vi "StateAlarmManagement.vi"(0 "Master State":enum16{"Normal", "Climb"}(ring)) -> ()   [LabVIEW 2020]
uses:
  sensordata.vi
  driverdata.vi
  autonomousinfo.vi
  robotoutputs.vi
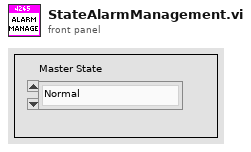
[diagram p1: front panel]
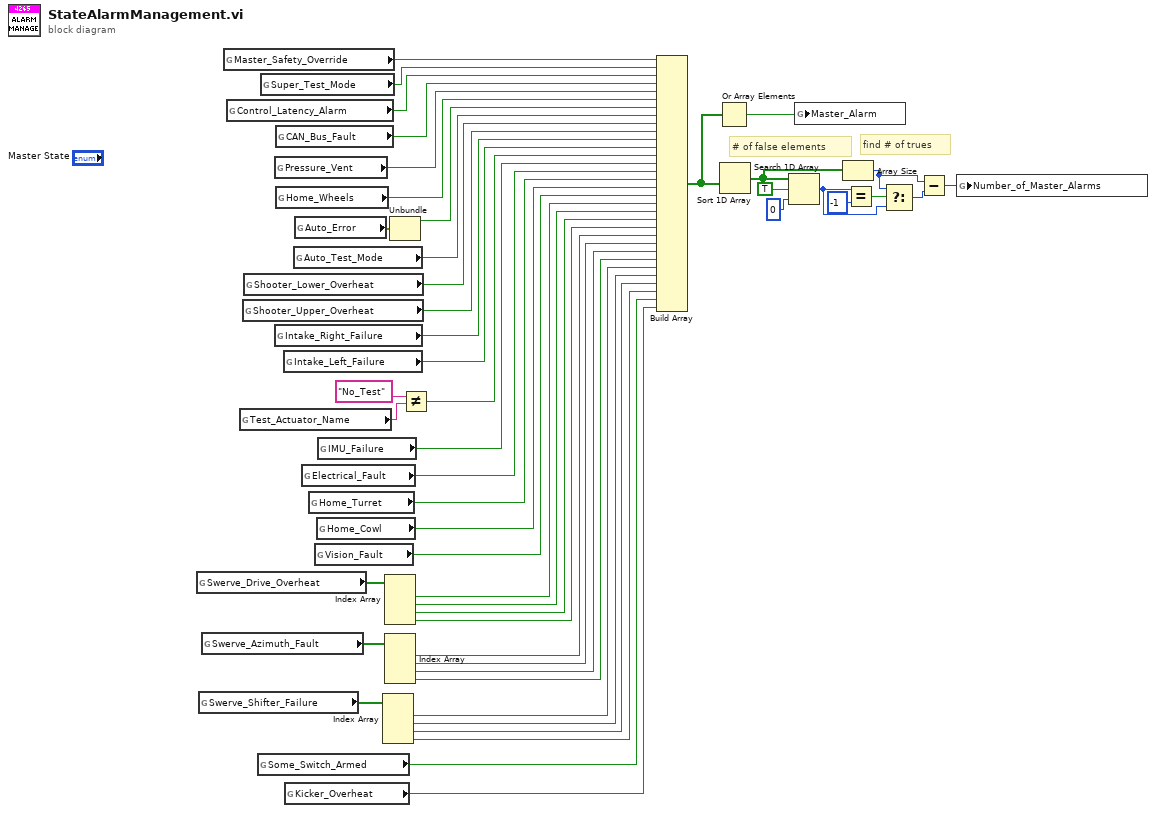
[diagram p0: block diagram]
diagram:
  # "# of false elements"
  # "find # of trues"
  n1 = global read "sensordata.vi" "Swerve_Drive_Overheat"() -> (w28:bool[])
  n2 = global read "sensordata.vi" "Swerve_Shifter_Failure"() -> (w18:bool[])
  n3 = global read "sensordata.vi" "Swerve_Azimuth_Fault"() -> (w23:bool[])
  n4 = global read "driverdata.vi" "Master_Safety_Override"() -> (w49:bool)
  n5 = global read "sensordata.vi" "Control_Latency_Alarm"() -> (w47:bool)
  n6 = global read "driverdata.vi" "Test_Actuator_Name"() -> (w37:string)
  n7 = global read "sensordata.vi" "Shooter_Upper_Overheat"() -> (w41:bool)
  n8 = global read "sensordata.vi" "Shooter_Lower_Overheat"() -> (w42:bool)
  n9 = global read "driverdata.vi" "Some_Switch_Armed"() -> (w13:bool)
  n10 = global read "driverdata.vi" "Super_Test_Mode"() -> (w48:bool)
  n11 = global read "sensordata.vi" "Pressure_Vent"() -> (w46:bool)
  n12 = global read "sensordata.vi" "Intake_Right_Failure"() -> (w40:bool)
  n13 = global read "sensordata.vi" "CAN_Bus_Fault"() -> (w33:bool)
  n14 = global read "driverdata.vi" "Home_Wheels"() -> (w32:bool)
  n15 = global read "sensordata.vi" "Intake_Left_Failure"() -> (w39:bool)
  n16 = global read "sensordata.vi" "Kicker_Overheat"() -> (w1:bool)
  n17 = global read "driverdata.vi" "Auto_Test_Mode"() -> (w43:bool)
  n18 = global read "autonomousinfo.vi" "Auto_Error"() -> (w45:errorcluster)
  n19 = global read "sensordata.vi" "Electrical_Fault"() -> (w34:bool)
  n20 = global read "driverdata.vi" "Home_Turret"() -> (w31:bool)
  n21 = global read "sensordata.vi" "Vision_Fault"() -> (w29:bool)
  n22 = global read "driverdata.vi" "Home_Cowl"() -> (w30:bool)
  n23 = global read "sensordata.vi" "IMU_Failure"() -> (w35:bool)
  n24 = Index Array(array=w18) -> (element #1=w17:bool, element #2=w16:bool, element #3=w15:bool, element #4=w14:bool)  [unwired: 4 in]
  n25 = Index Array(array=w28) -> (element #1=w27:bool, element #2=w26:bool, element #3=w25:bool, element #4=w24:bool)  [unwired: 4 in]
  n26 = Index Array(array=w23) -> (element #1=w22:bool, element #2=w21:bool, element #3=w20:bool, element #4=w19:bool)  [unwired: 4 in]
  n27 = Unbundle(w45) -> ("status"=w44:bool)  [unwired: 2 out]
  n28 = Not Equal?(x="No_Test", y=w37) -> (x != y?=w36:bool)
  n29 = Build Array(w49, w48, w47, w33, w46, w32, w44, w43, w42, w41, w40, w39, w36, w35, w34, w31, w30, w29, w27, w26, w25, w24, w22, w21, w20, w19, w17, w16, w15, w14, w13, w1) -> (w4:bool[])
  n30 = Or Array Elements(Boolean array=w4) -> (logical OR=w3:bool)
  n31 = Sort 1D Array(array=w4) -> (sorted array=w9:bool[])
  n32 = Search 1D Array(1D array=w9, element=TRUE, start index (0)=0) -> (index of element=w12:i32)
  n33 = global write "robotoutputs.vi" "Master_Alarm"(w3) -> ()
  n34 = Array Size(array=w9) -> (size(s)=w11:i32)
  n35 = Equal?(x=w12, y=-1) -> (x = y?=w8:bool)
  n36 = Select(t=w11, s=w8, f=w12) -> (s? t:f=w10:i32)
  n37 = Subtract(x=w11, y=w10) -> (x-y=w2:i32)
  n38 = global write "robotoutputs.vi" "Number_of_Master_Alarms"(w2) -> ()
